vi "Polarity switch 2 channel.vi"() -> ()   [LabVIEW 2017]
uses:
  <vilib>/DAQmx/write.llb/DAQmx Write (Digital 1D Bool NChan 1Samp 1Line).vi
  <vilib>/DAQmx/read.llb/DAQmx Read (Analog DBL 1Chan 1Samp).vi
  <vilib>/DAQmx/miscellaneous.llb/DAQmx Fill In Error Info.vi
  <instrlib>/Keithley KE22xx Series/Keithley KE22xx Series.lvlib
  <instrlib>/Harvard Apparatus PHD Ultra Series/Harvard Apparatus PHD Ultra Series.lvlib
  <instrlib>/J-KEM Quad temperature control/J-KEM Quad temperature control.lvlib
panel:
  out "Channel 2 voltage (V)":dbl format="%0.3f"
  in  "Voltage control set 2 (V)":dbl=3.0 format="%.2f"
  in  "Channel 2 control":bool
  in  "Voltage control set 1 (V)":dbl=3.0 format="%.2f"
  in  "Channel 1 control":bool
  in  "Control voltage":bool
  out "Channel 1 voltage (V)":dbl format="%0.3f"
  in  "Voltage set 2 (V)":dbl=3.0 format="%.3f"
  in  "Enable Output 2":bool
  in  "DC channel 2":bool
  out "Current 2 (mA)":dbl
  out "Voltage 2 (V)":dbl
  in  "Read voltage 2":bool
  in  "DC channel 1":bool
  in  "Target wait time 2 (min)":dbl
  in  "Count down 2":bool
  in  "New sample 2":bool
  in  "base path 2":path
  in  "Sample name 2":string
  in  "Stop&Save 2":bool
  in  "Saving data 2":bool
  in  "Start switching 2":bool
  in  "Switching time 2 (s)":dbl
  out "Present 2 (s)":dbl caption="Present (s)"
  out "Current time 2":timestamp
  out "Sample waiting time 2 (min)":dbl
  out "Start time 2":timestamp
  in  "Timing 2":bool
  in  "Channel 2 SP (C)":dbl format="%#_13g"
  in  "Channel 1 SP (C)":dbl format="%#_13g"
  out "Temperature plot":T1(graph)
  in  "Channel 2":bool
  out "Channel 2 temperature (C)":dbl
  out "Channel 1 temperature (C)":dbl
  in  "Channel 1":bool
  in  "J-KEM COM":refnum<visa-resource-name>="COM15"
  in  "Pump COM 2":refnum<visa-resource-name>="COM12"
  in  "Flow Rate (ul/min) 2":dbl=5.0 format="%#.4f"
  in  "Set flow 2":bool
  out "Infusing  2":bool
  out "Withdrawing 2":bool
  out "Idle 2":bool
  in  "Status 2":bool
  in  "Start 2":bool
  in  "Stop 2":bool
  out "Volume 2":dbl
  out "Volume Units 2":u16(ring) items=["milliliters", "microliters", "nanoliters", "picoliters"]
  in  "Read volume&time 2":bool
  in  "Set pump 2":bool
  out "error out 2":errorcluster
  in  "Read volume&time 1":bool
  out "Volume Units 1":u16(ring) items=["milliliters", "microliters", "nanoliters", "picoliters"]
  out "Volume 1":dbl
  in  "Set pump 1":bool
  in  "Stop 1":bool
  in  "Start 1":bool
  in  "Status 1":bool
  out "Infusing 1":bool
  out "Withdrawing 1":bool
  out "Idle 1":bool
  in  "Set flow 1":bool
  in  "Flow Rate (ul/min)":dbl=5.0 format="%#.4f"
  in  "Pump COM 1":refnum<visa-resource-name>="COM4"
  in  "Target wait time 1 (min)":dbl
  in  "Count down 1":bool
  in  "New sample 1":bool
  in  "Sample name 1":string
  in  "base path 1":path
  in  "Stop&Save 1":bool
  in  "Saving data 1":bool
  out "Sample waiting time 1 (min)":dbl
  out "Current time 1":timestamp
  out "Start time 1":timestamp
  in  "Timing 1":bool
  in  "Read voltage 1":bool
  out "Electrolysis current Chart":cluster{dbl, dbl}(graph)
  out "Voltage 1 (V)":dbl
  out "Current 1 (mA)":dbl
  in  "Voltage set 1 (V)":dbl=3.0 min=0.0 format="%.3f"
  in  "Enable Output 1":bool
  in  "DC power supply":refnum<visa-resource-name>="USB0::0x05E6::0x2230::9101650::INSTR"
  out "Present 1 (s)":dbl caption="Present (s)"
  in  "stop":bool
  in  "Switching time 1 (s)":dbl
  in  "Start switching 1":bool
  # "Temperature control"
  # "General settings"
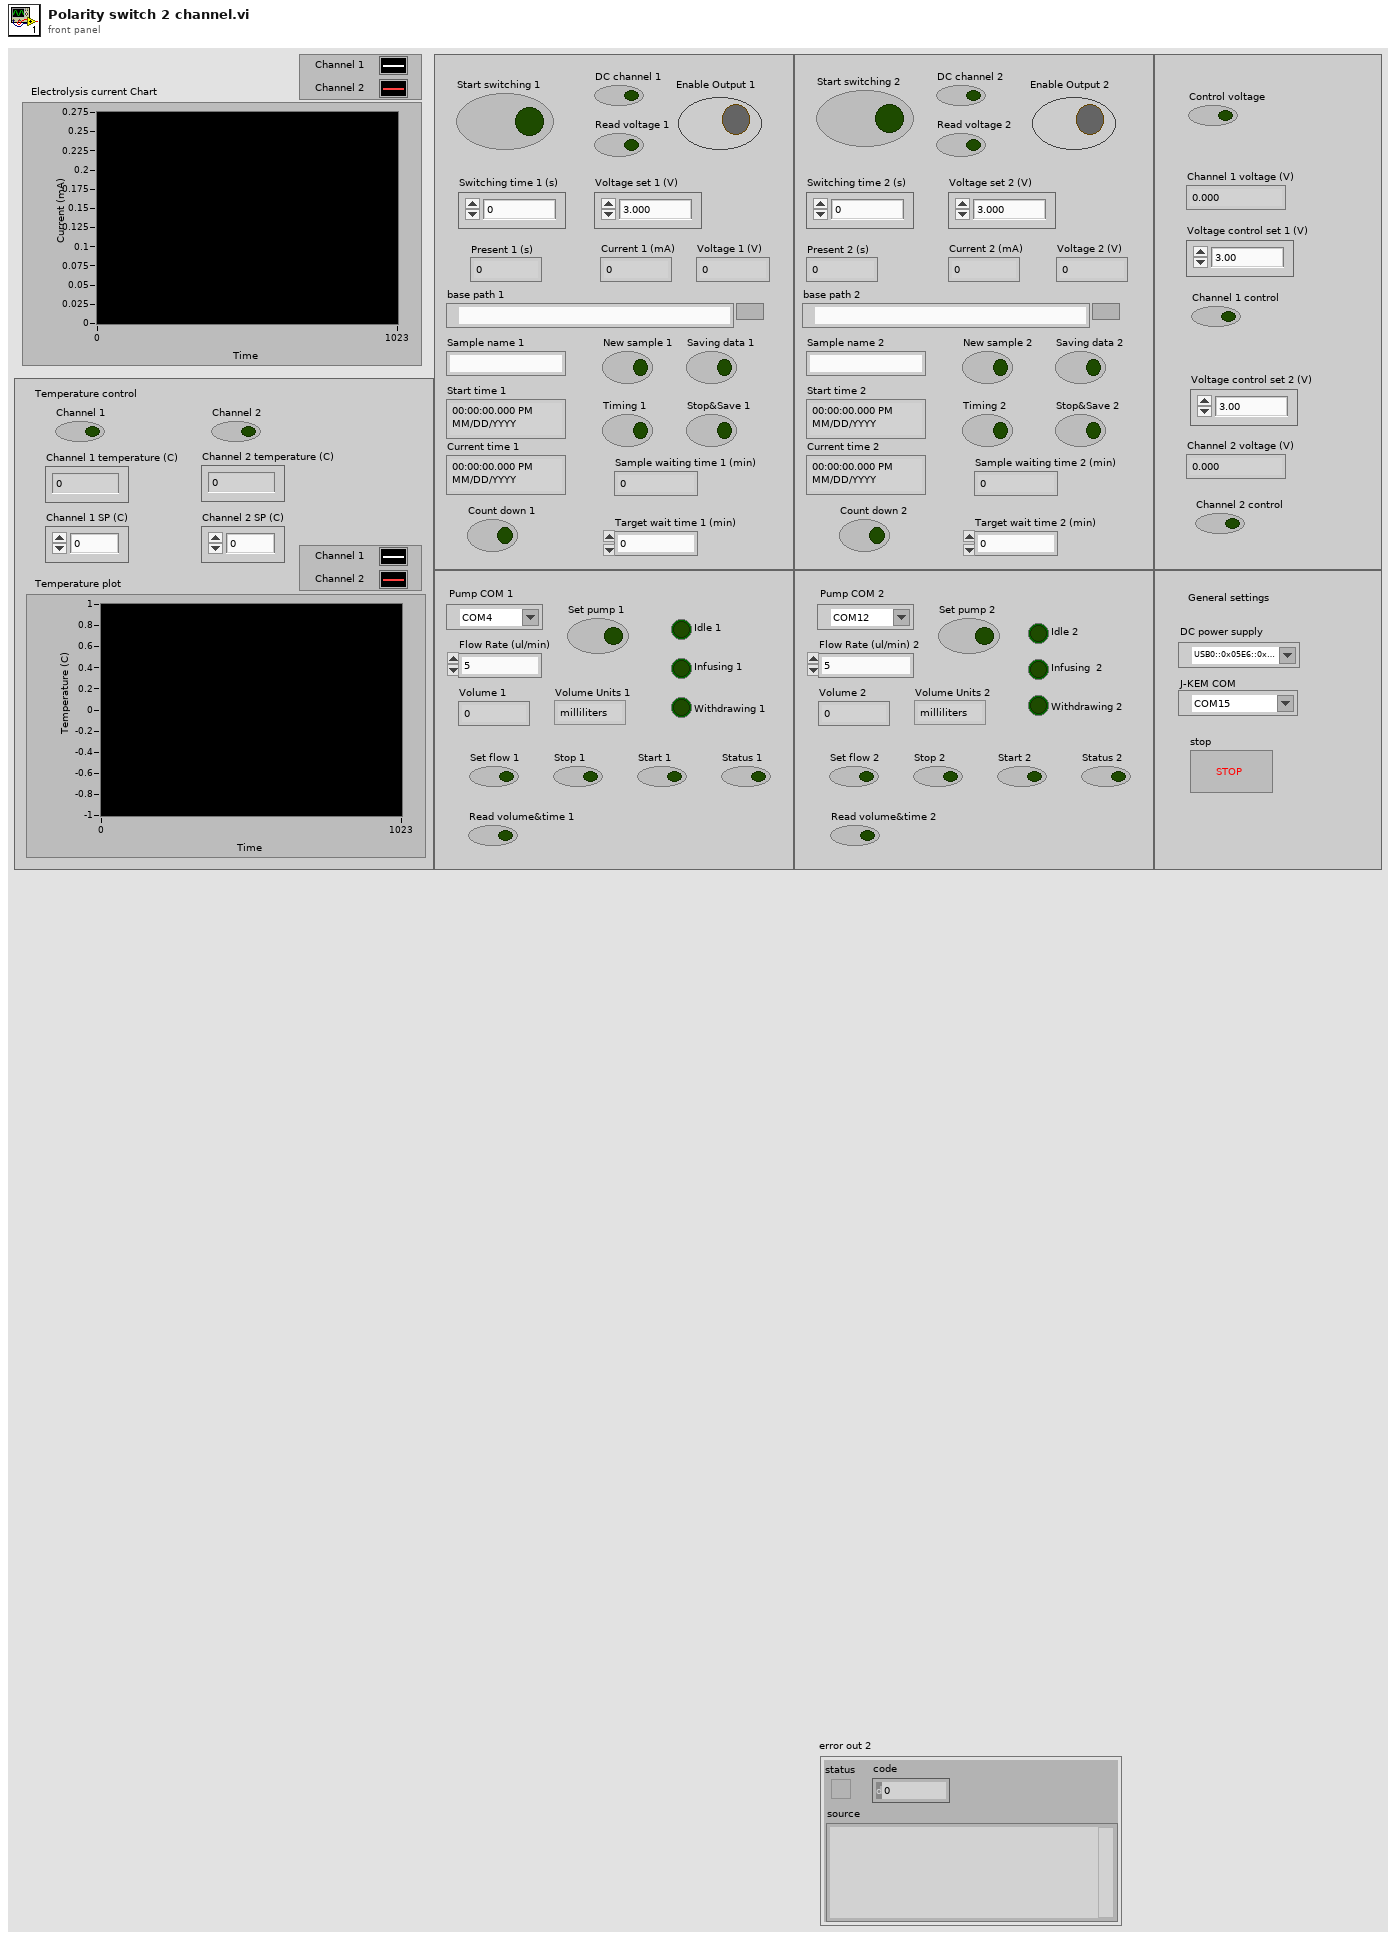
[diagram p1: front panel]
types:
  T1 = cluster{"Temperature (C)":dbl, "Temperature (C)":dbl}
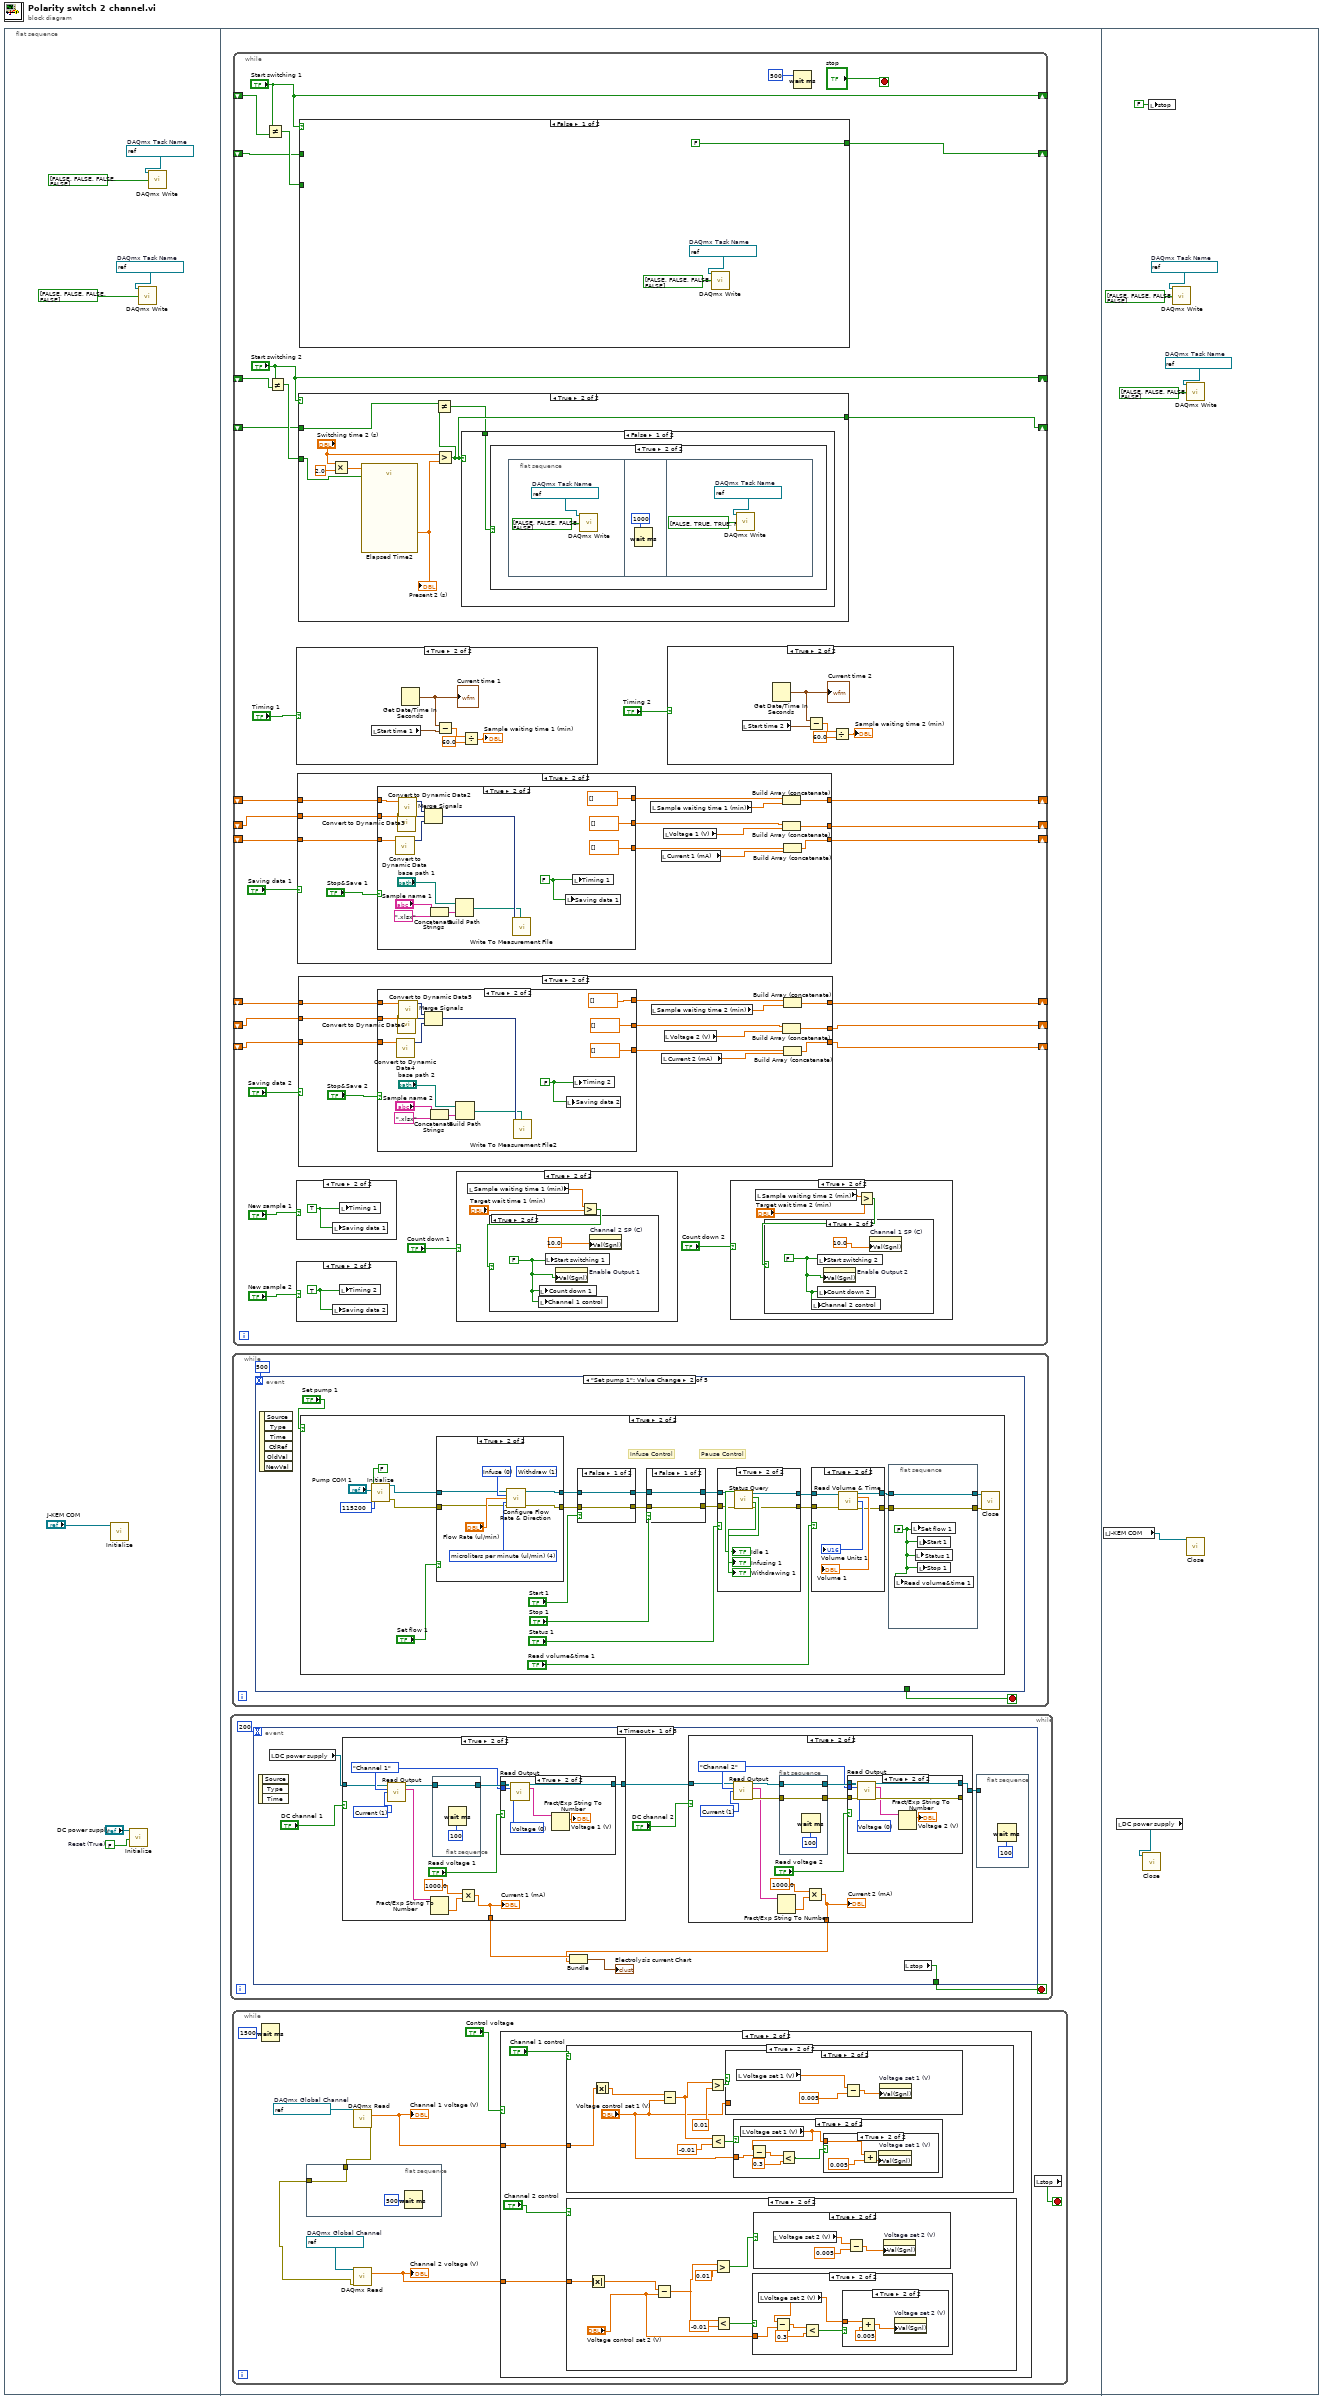
[diagram p0: block diagram]
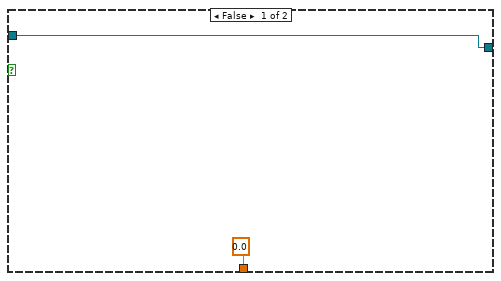
[diagram p11: hidden frame]
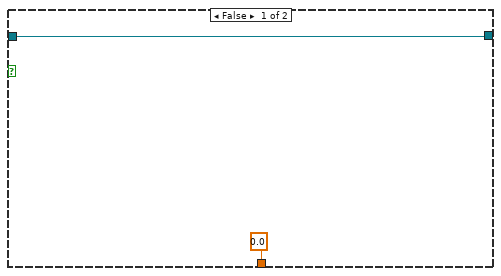
[diagram p13: hidden frame]
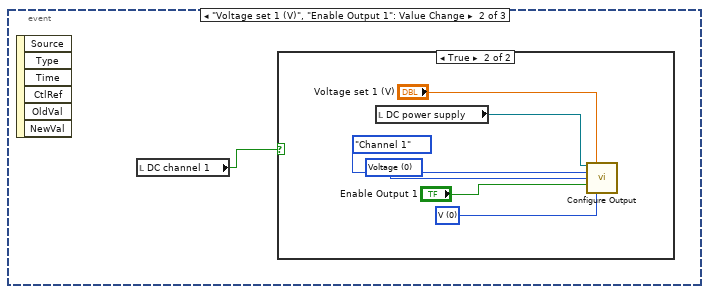
[diagram p15: hidden frame]
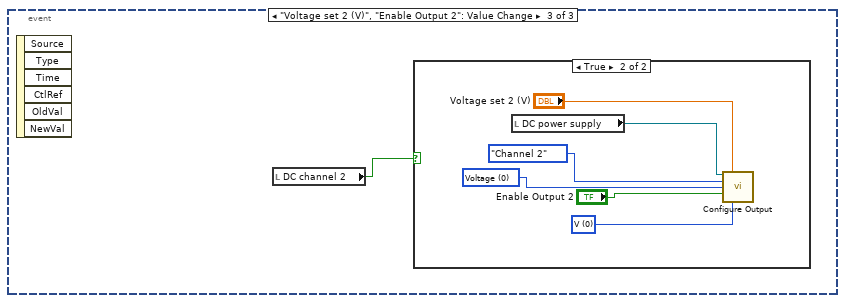
[diagram p17: hidden frame]
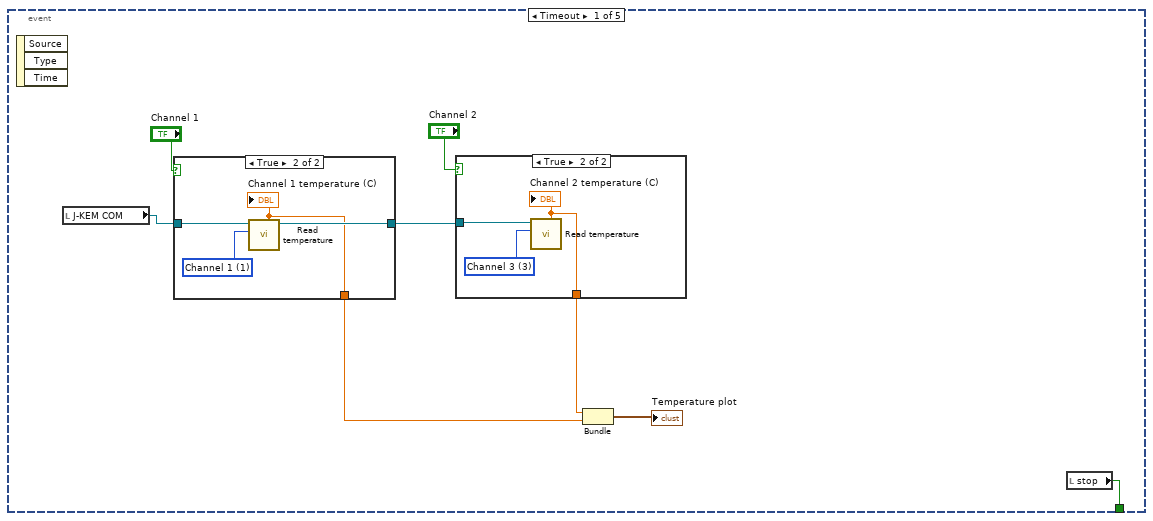
[diagram p19: hidden frame]
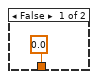
[diagram p20: hidden frame]
diagram:
  n1 = flat-sequence {
    frame #0 {
      w1 = refnum<k21> "Polarity swtich 2"  # DAQmx Task Name
      w5 = FALSE items=["OFF", "ON", "OFF", "ON"]  # Reset (True)
      w7 = refnum<k21> "Polarity switch 1"  # DAQmx Task Name
      n2 = call <instrlib>:"Initialize.vi"("VISA resource name"="J-KEM COM") -> ()  [unwired: 9 in, 2 out]
      n3 = call <instrlib>:"Initialize.vi"("Reset (True)"=w5, "VISA resource name"="DC power supply") -> ()  [unwired: 8 in, 2 out]
      n4 = call-poly <vilib>:"DAQmx Write.vi"("task/channels in"=w1, "data"=bool[] [FALSE, FALSE, FALSE, FALSE]) -> ()  [unwired: 11 in, 3 out]
      n5 = call-poly <vilib>:"DAQmx Write.vi"("task/channels in"=w7, "data"=bool[] [FALSE, FALSE, FALSE, FALSE]) -> ()  [unwired: 11 in, 3 out]
    }
    frame #1 {
      n6 = while {
        stop <- w62 stop-if-true
        n7 = event shown="[0] Timeout" {
          selector: _ -> [_ _ _]
          dyn-events: _ -> [_ _ _]
          timeout: 200 -> [_ _ _]
          tunnel: [w71 _ _] -> w62
          event Timeout {
            n8 = event-data() -> ()  [unwired: 1 in, 3 out]
            n9 = local read "DC power supply"() -> (w69:refnum<visa-resource-name>)
            n10 = case shown="True" "DC channel 1" {
              tunnel: w69 -> [w102 w105]
              tunnel: [w102 w104] -> w68
              tunnel: [0.0 w103] -> w66
              frame False {
              }
              frame True {
                w106 = u16 1 items=["Voltage", "Current", "Power"] ("Measurement Function (0:Voltage)")
                w108 = enum16{"Channel 1", "Channel 2", "Channel 3"}."Channel 1" ("Channel Select")
                n11 = call <instrlib>:"Read Output.vi"("VISA resource name"=w105, "Channel Select"=w108, "Measurement Function (0:Voltage)"=w106) -> ("VISA resource name out"=w112:refnum<visa-resource-name>, "Measurement"=w109:string)  [unwired: 10 in, 1 out]
                n12 = Fract/Exp String To Number(string=w109) -> (number=w110:dbl)  [unwired: 3 in, 1 out]
                n13 = flat-sequence {
                  tunnel: [w122] -> w111
                  tunnel: w112 -> [w122]
                  frame #0 {
                    n14 = Wait (ms)(milliseconds to wait=u32 100) -> ()  [unwired: 1 out]
                  }
                }
                n15 = Multiply(x=1000.0, y=w110) -> (x*y=w103:dbl)
                "Current 1 (mA)" <- w103
                n16 = case shown="True" "Read voltage 1" {
                  tunnel: [w114 w119] -> w104
                  tunnel: w111 -> [w114 w118]
                  tunnel: w108 -> [_ w117]
                  frame False {
                  }
                  frame True {
                    w120 = u16 0 items=["Voltage", "Current", "Power"] ("Measurement Function (0:Voltage)")
                    n17 = call <instrlib>:"Read Output.vi"("VISA resource name"=w118, "Channel Select"=w117, "Measurement Function (0:Voltage)"=w120) -> ("VISA resource name out"=w119:refnum<visa-resource-name>, "Measurement"=w115:string)  [unwired: 10 in, 1 out]
                    n18 = Fract/Exp String To Number(string=w115) -> (number=→"Voltage 1 (V)":dbl)  [unwired: 3 in, 1 out]
                  }
                }
              }
            }
            n19 = case shown="True" "DC channel 2" {
              tunnel: w68 -> [w73 w77]
              tunnel: [0.0 w76] -> w65
              tunnel: [w73 w75] -> w63
              frame False {
              }
              frame True {
                w78 = u16 1 items=["Voltage", "Current", "Power"] ("Measurement Function (0:Voltage)")
                w80 = enum16{"Channel 1", "Channel 2", "Channel 3"}."Channel 2" ("Channel Select")
                n20 = call <instrlib>:"Read Output.vi"("VISA resource name"=w77, "Channel Select"=w80, "Measurement Function (0:Voltage)"=w78) -> ("VISA resource name out"=w84:refnum<visa-resource-name>, "Measurement"=w81:string, "error out"=w86:errorcluster)  [unwired: 10 in]
                n21 = Fract/Exp String To Number(string=w81) -> (number=w82:dbl)  [unwired: 3 in, 1 out]
                n22 = flat-sequence {
                  tunnel: [w100] -> w83
                  tunnel: w84 -> [w100]
                  tunnel: [w99] -> w85
                  tunnel: w86 -> [w99]
                  frame #0 {
                    n23 = Wait (ms)(milliseconds to wait=u32 100) -> ()  [unwired: 1 out]
                  }
                }
                n24 = Multiply(x=1000.0, y=w82) -> (x*y=w76:dbl)
                "Current 2 (mA)" <- w76
                n25 = case shown="True" "Read voltage 2" {
                  tunnel: [w89 w96] -> w75
                  tunnel: [w88 w95] -> _
                  tunnel: w83 -> [w89 w94]
                  tunnel: w85 -> [w88 w93]
                  tunnel: w80 -> [_ w92]
                  frame False {
                  }
                  frame True {
                    w97 = u16 0 items=["Voltage", "Current", "Power"] ("Measurement Function (0:Voltage)")
                    n26 = call <instrlib>:"Read Output.vi"("VISA resource name"=w94, "Channel Select"=w92, "Measurement Function (0:Voltage)"=w97, "error in (no error)"=w93) -> ("VISA resource name out"=w96:refnum<visa-resource-name>, "Measurement"=w90:string, "error out"=w95:errorcluster)  [unwired: 9 in]
                    n27 = Fract/Exp String To Number(string=w90) -> (number=→"Voltage 2 (V)":dbl)  [unwired: 3 in, 1 out]
                  }
                }
              }
            }
            n28 = Bundle(w66, w65) -> (→"Electrolysis current Chart":cluster{dbl, dbl})  [unwired: 1 in]
            n29 = local read "stop"() -> (w71:bool)
            n30 = flat-sequence {
              tunnel: w63 -> [_]
              frame #0 {
                n31 = Wait (ms)(milliseconds to wait=u32 100) -> ()  [unwired: 1 out]
              }
            }
          }
          event "Voltage set 1 (V)", "Enable Output 1": Value Change {
            n32 = event-data() -> ()  [unwired: 1 in, 6 out]
            n33 = local read "DC channel 1"() -> (w123:bool)
            n34 = case shown="True" w123 {
              frame False {
              }
              frame True {
                w125 = u16 0 items=["Voltage", "Current"] ("Function(0:Voltage)")
                w124 = u16 0 items=["V", "mV", "kV", "A", "mA"] ("Unit(V)")
                n35 = local read "DC power supply"() -> (w127:refnum<visa-resource-name>)
                n36 = call <instrlib>:"Configure Output.vi"("VISA resource name"=w127, "Manual Range(0.00)"="Voltage set 1 (V)", "Channel Select"=enum16{"Channel 1", "Channel 2", "Channel 3"}."Channel 1", "Function(0:Voltage)"=w125, "Enable Output (T: Enable)"="Enable Output 1", "Unit(V)"=w124) -> ()  [unwired: 8 in, 2 out]
              }
            }
          }
          event "Voltage set 2 (V)", "Enable Output 2": Value Change {
            n37 = event-data() -> ()  [unwired: 1 in, 6 out]
            n38 = local read "DC channel 2"() -> (w130:bool)
            n39 = case shown="True" w130 {
              frame False {
              }
              frame True {
                w132 = u16 0 items=["Voltage", "Current"] ("Function(0:Voltage)")
                w131 = u16 0 items=["V", "mV", "kV", "A", "mA"] ("Unit(V)")
                n40 = local read "DC power supply"() -> (w134:refnum<visa-resource-name>)
                n41 = call <instrlib>:"Configure Output.vi"("VISA resource name"=w134, "Manual Range(0.00)"="Voltage set 2 (V)", "Channel Select"=enum16{"Channel 1", "Channel 2", "Channel 3"}."Channel 2", "Function(0:Voltage)"=w132, "Enable Output (T: Enable)"="Enable Output 2", "Unit(V)"=w131) -> ()  [unwired: 8 in, 2 out]
              }
            }
          }
        }
      }
      n42 = while {
        stop <- w137 stop-if-true
        n43 = event shown="[1] \"Set pump 1\": Value Change" {
          selector: _ -> [_ _ _ _ _]
          dyn-events: _ -> [_ _ _ _ _]
          timeout: 500 -> [_ _ _ _ _]
          tunnel: [w139 _ _ _ _] -> w137
          event Timeout {
            n44 = event-data() -> ()  [unwired: 1 in, 3 out]
            n45 = local read "J-KEM COM"() -> (w145:refnum<visa-resource-name>)
            n46 = case shown="True" "Channel 1" {
              tunnel: w145 -> [w152 w156]
              tunnel: [w152 w154] -> w144
              tunnel: [0.0 ("Temperature (C)") w153] -> w142
              frame False {
              }
              frame True {
                w155 = u16 1 items=["Channel 1"=1, "Channel 2"=2, "Channel 3"=3, "Channel 4"=4] ("Channel")
                n47 = call <instrlib>:"Read temperature.vi"("Channel"=w155, "VISA resource"=w156) -> ("Temperature (C)"=w153:dbl, "VISA resource"=w154:refnum<visa-resource-name>)  [unwired: 7 in, 1 out]
                "Channel 1 temperature (C)" <- w153
              }
            }
            n48 = case shown="True" "Channel 2" {
              tunnel: w144 -> [_ w150]
              tunnel: [0.0 ("Temperature (C)") w148] -> w141
              frame False {
              }
              frame True {
                w149 = u16 3 items=["Channel 1"=1, "Channel 2"=2, "Channel 3"=3, "Channel 4"=4] ("Channel")
                n49 = call <instrlib>:"Read temperature.vi"("Channel"=w149, "VISA resource"=w150) -> ("Temperature (C)"=w148:dbl)  [unwired: 7 in, 2 out]
                "Channel 2 temperature (C)" <- w148
              }
            }
            n50 = Bundle("Temperature (C)"=w141, "Temperature (C)"=w142) -> (→"Temperature plot":T1)  [unwired: 1 in]
            n51 = local read "stop"() -> (w139:bool)
          }
          event "Set pump 1": Value Change {
            n52 = event-data() -> ()  [unwired: 1 in, 6 out]
            n53 = case shown="True" "Set pump 1" {
              frame False {
              }
              frame True {
                w178 = u32 115200 items=["9600"=9600, "19200"=19200, "38400"=38400, "57600"=57600, "115200"=115200] ("Baud Rate (115200)")
                # "Pause Control"
                # "Infuse Control"
                n54 = call <instrlib>:"Initialize.vi"("ID Query (True)"=FALSE, "Baud Rate (115200)"=w178, "VISA resource name"="Pump COM 1") -> ("error out"=w173:errorcluster, "VISA resource name out"=w174:refnum<visa-resource-name>)  [unwired: 7 in]
                n55 = case shown="True" "Set flow 1" {
                  tunnel: w174 -> [w201 w205]
                  tunnel: w173 -> [w200 w204]
                  tunnel: [w201 w203] -> w172
                  tunnel: [w200 w202] -> w171
                  frame False {
                  }
                  frame True {
                    w206 = u32 4 items=["milliliters per hour (ml/hr)", "milliliters per minute (ml/min)", "milliliters per second (ml/sec)", "microliters per hour (ul/hr)", "microliters per minute (ul/min)", "microliters per second (ul/sec)", "nanoliters per hour (nl/hr)", "nanoliters per minute (nl/min)", "nanoliters per second (nl/sec)", "picoliters per hour (pl/hr)", "picoliters per minute (pl/min)", "picoliters per second (pl/sec)"] ("Flow Rate Units")
                    w208 = u16 0 items=["Infuse", "Withdraw"] ("Pump Method (0:Infuse)")
                    (unwired) u16 1 items=["Infuse", "Withdraw"] ("Pump Method (0:Infuse)")
                    n56 = call <instrlib>:"Configure Flow Rate & Direction.vi"("VISA resource name"=w205, "Pump Direction (0:Infuse)"=w208, "Flow Rate (5.00)"="Flow Rate (ul/min)", "Flow Rate Units (1:ml/min)"=w206, "error in (no error)"=w204) -> ("VISA resource name out"=w203:refnum<visa-resource-name>, "error out"=w202:errorcluster)  [unwired: 9 in]
                  }
                }
                n57 = case shown="False" "Start 1" {
                  tunnel: [w216 w221] -> w177
                  tunnel: [w215 w220] -> w176
                  tunnel: w172 -> [w216 w218]
                  tunnel: w171 -> [w215 w217]
                  frame False {
                  }
                  frame True {
                    w219 = u16 0 items=["Infuse", "Withdraw"] ("Run Method (0:Infuse)")
                    n58 = call <instrlib>:"Start Pump.vi"("error in (no error)"=w217, "Run Direction (0:Infuse)"=w219, "VISA resource name"=w218) -> ("error out"=w220:errorcluster, "VISA resource name out"=w221:refnum<visa-resource-name>)  [unwired: 7 in]
                  }
                }
                n59 = case shown="False" "Stop 1" {
                  tunnel: w177 -> [w210 w214]
                  tunnel: w176 -> [w209 w213]
                  tunnel: [w210 w212] -> w170
                  tunnel: [w209 w211] -> w169
                  frame False {
                  }
                  frame True {
                    n60 = call <instrlib>:"Stop Pump.vi"("error in (no error)"=w213, "VISA resource name"=w214) -> ("error out"=w211:errorcluster, "VISA resource name out"=w212:refnum<visa-resource-name>)  [unwired: 8 in]
                  }
                }
                n61 = case shown="True" "Status 1" {
                  tunnel: w170 -> [w192 w196]
                  tunnel: w169 -> [w191 w195]
                  tunnel: [w192 w194] -> w162
                  tunnel: [w191 w193] -> w161
                  frame False {
                  }
                  frame True {
                    n62 = call <instrlib>:"Status Query.vi"("error in (no error)"=w195, "VISA resource name"=w196) -> ("error out"=w193:errorcluster, "Withdrawing"=→"Withdrawing 1":bool, "Infusing"=→"Infusing 1":bool, "VISA resource name out"=w194:refnum<visa-resource-name>, "Idle"=→"Idle 1":bool)  [unwired: 4 in, 1 out]
                  }
                }
                n63 = case shown="True" "Read volume&time 1" {
                  tunnel: w162 -> [w181 w187]
                  tunnel: w161 -> [w180 w186]
                  tunnel: [w181 w183] -> w160
                  tunnel: [w180 w182] -> w159
                  frame False {
                  }
                  frame True {
                    n64 = call <instrlib>:"Read Volume & Time .vi"("VISA resource name"=w187, "error in (no error)"=w186) -> ("VISA resource name out"=w183:refnum<visa-resource-name>, "Volume"=→"Volume 1":dbl, "Volume Units"=→"Volume Units 1":u16, "error out"=w182:errorcluster)  [unwired: 8 in, 2 out]
                  }
                }
                n65 = flat-sequence {
                  tunnel: w160 -> [w189]
                  tunnel: [w190] -> w165
                  tunnel: w159 -> [w190]
                  tunnel: [w189] -> w164
                  frame #0 {
                    w188 = FALSE
                    n66 = local write "Read volume&time 1"(w188) -> ()
                    n67 = local write "Set flow 1"(w188) -> ()
                    n68 = local write "Status 1"(w188) -> ()
                    n69 = local write "Start 1"(w188) -> ()
                    n70 = local write "Stop 1"(w188) -> ()
                  }
                }
                n71 = call <instrlib>:"Close.vi"("error in (no error)"=w165, "VISA resource name"=w164) -> ()  [unwired: 9 in, 1 out]
              }
            }
          }
          event "Set pump 2": Value Change {
            n72 = event-data() -> ()  [unwired: 1 in, 6 out]
            n73 = case shown="True" "Set pump 2" {
              frame False {
              }
              frame True {
                w243 = u32 115200 items=["9600"=9600, "19200"=19200, "38400"=38400, "57600"=57600, "115200"=115200] ("Baud Rate (115200)")
                # "Pause Control"
                # "Infuse Control"
                n74 = call <instrlib>:"Initialize.vi"("ID Query (True)"=FALSE, "Baud Rate (115200)"=w243, "VISA resource name"="Pump COM 2") -> ("error out"=w238:errorcluster, "VISA resource name out"=w239:refnum<visa-resource-name>)  [unwired: 7 in]
                "error out 2" <- w238
                n75 = case shown="True" "Set flow 2" {
                  tunnel: w239 -> [w266 w270]
                  tunnel: w238 -> [w265 w269]
                  tunnel: [w266 w268] -> w237
                  tunnel: [w265 w267] -> w236
                  frame False {
                  }
                  frame True {
                    w271 = u32 4 items=["milliliters per hour (ml/hr)", "milliliters per minute (ml/min)", "milliliters per second (ml/sec)", "microliters per hour (ul/hr)", "microliters per minute (ul/min)", "microliters per second (ul/sec)", "nanoliters per hour (nl/hr)", "nanoliters per minute (nl/min)", "nanoliters per second (nl/sec)", "picoliters per hour (pl/hr)", "picoliters per minute (pl/min)", "picoliters per second (pl/sec)"] ("Flow Rate Units")
                    w273 = u16 0 items=["Infuse", "Withdraw"] ("Pump Method (0:Infuse)")
                    (unwired) u16 1 items=["Infuse", "Withdraw"] ("Pump Method (0:Infuse)")
                    n76 = call <instrlib>:"Configure Flow Rate & Direction.vi"("VISA resource name"=w270, "Pump Direction (0:Infuse)"=w273, "Flow Rate (5.00)"="Flow Rate (ul/min) 2", "Flow Rate Units (1:ml/min)"=w271, "error in (no error)"=w269) -> ("VISA resource name out"=w268:refnum<visa-resource-name>, "error out"=w267:errorcluster)  [unwired: 9 in]
                  }
                }
                n77 = case shown="False" "Start 2" {
                  tunnel: [w281 w286] -> w242
                  tunnel: [w280 w285] -> w241
                  tunnel: w237 -> [w281 w283]
                  tunnel: w236 -> [w280 w282]
                  frame False {
                  }
                  frame True {
                    w284 = u16 0 items=["Infuse", "Withdraw"] ("Run Method (0:Infuse)")
                    n78 = call <instrlib>:"Start Pump.vi"("error in (no error)"=w282, "Run Direction (0:Infuse)"=w284, "VISA resource name"=w283) -> ("error out"=w285:errorcluster, "VISA resource name out"=w286:refnum<visa-resource-name>)  [unwired: 7 in]
                  }
                }
                n79 = case shown="False" "Stop 2" {
                  tunnel: w242 -> [w275 w279]
                  tunnel: w241 -> [w274 w278]
                  tunnel: [w275 w277] -> w235
                  tunnel: [w274 w276] -> w234
                  frame False {
                  }
                  frame True {
                    n80 = call <instrlib>:"Stop Pump.vi"("error in (no error)"=w278, "VISA resource name"=w279) -> ("error out"=w276:errorcluster, "VISA resource name out"=w277:refnum<visa-resource-name>)  [unwired: 8 in]
                  }
                }
                n81 = case shown="True" "Status 2" {
                  tunnel: w235 -> [w257 w261]
                  tunnel: w234 -> [w256 w260]
                  tunnel: [w257 w259] -> w227
                  tunnel: [w256 w258] -> w226
                  frame False {
                  }
                  frame True {
                    n82 = call <instrlib>:"Status Query.vi"("error in (no error)"=w260, "VISA resource name"=w261) -> ("error out"=w258:errorcluster, "Withdrawing"=→"Withdrawing 2":bool, "Infusing"=→"Infusing  2":bool, "VISA resource name out"=w259:refnum<visa-resource-name>, "Idle"=→"Idle 2":bool)  [unwired: 4 in, 1 out]
                  }
                }
                n83 = case shown="True" "Read volume&time 2" {
                  tunnel: w227 -> [w246 w252]
                  tunnel: w226 -> [w245 w251]
                  tunnel: [w246 w248] -> w225
                  tunnel: [w245 w247] -> w224
                  frame False {
                  }
                  frame True {
                    n84 = call <instrlib>:"Read Volume & Time .vi"("VISA resource name"=w252, "error in (no error)"=w251) -> ("VISA resource name out"=w248:refnum<visa-resource-name>, "Volume"=→"Volume 2":dbl, "Volume Units"=→"Volume Units 2":u16, "error out"=w247:errorcluster)  [unwired: 8 in, 2 out]
                  }
                }
                n85 = flat-sequence {
                  tunnel: w225 -> [w254]
                  tunnel: [w255] -> w230
                  tunnel: w224 -> [w255]
                  tunnel: [w254] -> w229
                  frame #0 {
                    w253 = FALSE
                    n86 = local write "Read volume&time 2"(w253) -> ()
                    n87 = local write "Set flow 2"(w253) -> ()
                    n88 = local write "Status 2"(w253) -> ()
                    n89 = local write "Start 2"(w253) -> ()
                    n90 = local write "Stop 2"(w253) -> ()
                  }
                }
                n91 = call <instrlib>:"Close.vi"("error in (no error)"=w230, "VISA resource name"=w229) -> ()  [unwired: 9 in, 1 out]
              }
            }
          }
          event "Channel 1 SP (C)": Value Change {
            n92 = event-data() -> ()  [unwired: 1 in, 6 out]
            n93 = local read "Channel 1"() -> (w287:bool)
            n94 = case shown="True" w287 {
              frame False {
              }
              frame True {
                w289 = u16 1 items=["Channel 1"=1, "Channel 2"=2, "Channel 3"=3, "Channel 4"=4] ("Channel")
                n95 = local read "J-KEM COM"() -> (w290:refnum<visa-resource-name>)
                n96 = call <instrlib>:"Set SP.vi"("Set point (C)"="Channel 1 SP (C)", "Channel"=w289, "VISA resource name"=w290) -> ()  [unwired: 6 in, 3 out]
                n97 = Wait (ms)(milliseconds to wait=u32 1000) -> ()  [unwired: 1 out]
              }
            }
          }
          event "Channel 2 SP (C)": Value Change {
            n98 = event-data() -> ()  [unwired: 1 in, 6 out]
            n99 = local read "Channel 2"() -> (w292:bool)
            n100 = case shown="True" w292 {
              frame False {
              }
              frame True {
                w294 = u16 3 items=["Channel 1"=1, "Channel 2"=2, "Channel 3"=3, "Channel 4"=4] ("Channel")
                n101 = local read "J-KEM COM"() -> (w296:refnum<visa-resource-name>)
                n102 = call <instrlib>:"Set SP.vi"("Set point (C)"="Channel 2 SP (C)", "Channel"=w294, "VISA resource name"=w296) -> ()  [unwired: 6 in, 3 out]
                n103 = Wait (ms)(milliseconds to wait=u32 1000) -> ()  [unwired: 1 out]
              }
            }
          }
        }
      }
      n104 = while {
        stop <- w16 stop-if-true
        w11 = refnum<k21> "USB-6221 ai1"  # DAQmx Global Channel
        w13 = refnum<k21> "USB-6221 ai0"  # DAQmx Global Channel
        n105 = Wait (ms)(milliseconds to wait=u32 1500) -> ()  [unwired: 1 out]
        n106 = flat-sequence {
          tunnel: w10 -> [w18]
          tunnel: [w18] -> w9
          frame #0 {
            n107 = Wait (ms)(milliseconds to wait=u32 500) -> ()  [unwired: 1 out]
          }
        }
        n108 = call-poly <vilib>:"DAQmx Read.vi"("task/channels in"=w13) -> ("data"=w12:dbl, "error out"=w10:errorcluster)  [unwired: 12 in, 1 out]
        "Channel 1 voltage (V)" <- w12
        n109 = call-poly <vilib>:"DAQmx Read.vi"("task/channels in"=w11, "error in"=w9) -> ("data"=w8:dbl)  [unwired: 11 in, 2 out]
        "Channel 2 voltage (V)" <- w8
        n110 = case shown="True" "Control voltage" {
          tunnel: w12 -> [_ w21]
          tunnel: w8 -> [_ w19]
          frame False {
          }
          frame True {
            n111 = case shown="True" "Channel 1 control" {
              tunnel: w21 -> [_ w43]
              frame False {
              }
              frame True {
                n112 = Absolute Value(x=w43) -> (abs(x)=w49:dbl)
                n113 = Subtract(x=w49, y="Voltage control set 1 (V)") -> (x-y=w46:dbl)
                n114 = Greater?(x=w46, y=0.01) -> (0:w47:bool)
                n115 = Less?(x=w46, y=-0.01) -> (x < y?=w44:bool)
                n116 = case shown="True" w47 {
                  tunnel: "Voltage control set 1 (V)" -> [_ _]
                  frame False {
                  }
                  frame True {
                    n117 = local read "Voltage set 1 (V)"() -> (w60:dbl)
                    n118 = Subtract(x=w60, y=0.005) -> (x-y=w58:dbl)
                    n119 = property on="Voltage set 1 (V)" class="DigNum (strict)"("Val(Sgnl)"=w58) -> ()  [unwired: 2 in, 2 out]
                  }
                }
                n120 = case shown="True" w44 {
                  tunnel: "Voltage control set 1 (V)" -> [_ w54]
                  frame False {
                  }
                  frame True {
                    n121 = local read "Voltage set 1 (V)"() -> (w53:dbl)
                    n122 = Subtract(x=w53, y=w54) -> (x-y=w50:dbl)
                    n123 = Less?(x=w50, y=0.3) -> (x < y?=w51:bool)
                    n124 = case shown="True" w51 {
                      tunnel: w53 -> [_ w55]
                      frame False {
                      }
                      frame True {
                        n125 = Add(x=w55, y=0.005) -> (x+y=w56:dbl)
                        n126 = property on="Voltage set 1 (V)" class="DigNum (strict)"("Val(Sgnl)"=w56) -> ()  [unwired: 2 in, 2 out]
                      }
                    }
                  }
                }
              }
            }
            n127 = case shown="True" "Channel 2 control" {
              tunnel: w19 -> [_ w30]
              frame False {
              }
              frame True {
                n128 = Absolute Value(x=w30) -> (abs(x)=w29:dbl)
                n129 = Subtract(x=w29, y="Voltage control set 2 (V)") -> (x-y=w26:dbl)
                n130 = Greater?(x=w26, y=0.01) -> (0:w25:bool)
                n131 = Less?(x=w26, y=-0.01) -> (x < y?=w24:bool)
                n132 = case shown="True" w24 {
                  tunnel: "Voltage control set 2 (V)" -> [_ w33]
                  frame False {
                  }
                  frame True {
                    n133 = local read "Voltage set 2 (V)"() -> (w32:dbl)
                    n134 = Subtract(x=w32, y=w33) -> (x-y=w35:dbl)
                    n135 = Less?(x=w35, y=0.3) -> (x < y?=w31:bool)
                    n136 = case shown="True" w31 {
                      tunnel: w32 -> [_ w36]
                      frame False {
                      }
                      frame True {
                        n137 = Add(x=w36, y=0.005) -> (x+y=w37:dbl)
                        n138 = property on="Voltage set 2 (V)" class="DigNum (strict)"("Val(Sgnl)"=w37) -> ()  [unwired: 2 in, 2 out]
                      }
                    }
                  }
                }
                n139 = case shown="True" w25 {
                  frame False {
                  }
                  frame True {
                    n140 = local read "Voltage set 2 (V)"() -> (w40:dbl)
                    n141 = Subtract(x=w40, y=0.005) -> (x-y=w39:dbl)
                    n142 = property on="Voltage set 2 (V)" class="DigNum (strict)"("Val(Sgnl)"=w39) -> ()  [unwired: 2 in, 2 out]
                  }
                }
              }
            }
          }
        }
        n143 = local read "stop"() -> (w16:bool)
      }
      n144 = while {
        shift-right: ["Start switching 1"] -> _
        shift-left: _ -> [w327]
        shift-right: [w325] -> _
        shift-left: _ -> [w324]
        shift-right: [w319] -> _
        shift-left: _ -> [w317]
        shift-right: [w318] -> _
        shift-left: _ -> [w316]
        shift-right: ["Start switching 2"] -> _
        shift-left: _ -> [w311]
        shift-right: [w309] -> _
        shift-left: _ -> [w308]
        shift-right: [w307] -> _
        shift-left: _ -> [w306]
        shift-right: [w304] -> _
        shift-left: _ -> [w301]
        shift-right: [w303] -> _
        shift-left: _ -> [w300]
        shift-right: [w302] -> _
        shift-left: _ -> [w299]
        stop <- "stop" stop-if-true
        n145 = Not Equal?(x="Start switching 1", y=w327) -> (x != y?=w326:bool)
        n146 = Not Equal?(x="Start switching 2", y=w311) -> (x != y?=w310:bool)
        n147 = case shown="True" "Timing 1" {
          frame False {
            n148 = Get Date/Time In Seconds() -> (seconds since 1Jan1904=→"Start time 1":timestamp)
          }
          frame True {
            n149 = local read "Start time 1"() -> (w444:timestamp)
            n150 = Get Date/Time In Seconds() -> (seconds since 1Jan1904=w445:timestamp)
            "Current time 1" <- w445
            n151 = Subtract(x=w445, y=w444) -> (x-y=w442:dbl)
            n152 = Divide(x=w442, y=60.0) -> (x/y=→"Sample waiting time 1 (min)":dbl)
          }
        }
        n153 = case shown="True" "New sample 1" {
          frame False {
          }
          frame True {
            w404 = TRUE ("Timing")
            n154 = local write "Saving data 1"(w404) -> ()
            n155 = local write "Timing 1"(w404) -> ()
          }
        }
        n156 = case shown="True" "New sample 2" {
          frame False {
          }
          frame True {
            w334 = TRUE ("Timing")
            n157 = local write "Saving data 2"(w334) -> ()
            n158 = local write "Timing 2"(w334) -> ()
          }
        }
        n159 = case shown="True" "Saving data 1" {
          tunnel: [dbl[] [] w420] -> w319
          tunnel: [dbl[] [] w412] -> w318
          tunnel: w317 -> [_ w415]
          tunnel: w316 -> [_ w414]
          tunnel: [dbl[] [] w409] -> w307
          tunnel: w306 -> [_ w408]
          frame False {
          }
          frame True {
            n160 = case shown="True" "Stop&Save 1" {
              tunnel: [w423 dbl[] []] -> w416
              tunnel: w415 -> [w423 w438]
              tunnel: [w421 dbl[] []] -> w410
              tunnel: w414 -> [w422 w439]
              tunnel: [w422 dbl[] []] -> w411
              tunnel: w408 -> [w421 w426]
              frame False {
              }
              frame True {
                w428 = FALSE ("Timing")
                n161 = call "Convert to Dynamic Data"("Array"=w439) -> ("Dynamic Data Type"=w424:dynamicdata)  [unwired: 3 in]
                n162 = call "Convert to Dynamic Data3"("Array"=w426) -> ("Dynamic Data Type"=w425:dynamicdata)  [unwired: 3 in]
                n163 = call "Convert to Dynamic Data2"("Array"=w438) -> ("Dynamic Data Type"=w437:dynamicdata)  [unwired: 3 in]
                n164 = Merge Signals(w437, w425, w424) -> (w436:dynamicdata)
                n165 = Concatenate Strings("Sample name 1", ".xlsx" ("string")) -> (w430:string)
                n166 = Build Path(base path="base path 1", name or relative path=w430) -> (appended path=w434:path)
                n167 = call "Write To Measurement File"("Signals"=w436, "Filename"=w434) -> ()  [unwired: 15 in, 3 out]
                n168 = local write "Saving data 1"(w428) -> ()
                n169 = local write "Timing 1"(w428) -> ()
              }
            }
            n170 = local read "Sample waiting time 1 (min)"() -> (w419:dbl)
            n171 = local read "Current 1 (mA)"() -> (w418:dbl)
            n172 = local read "Voltage 1 (V)"() -> (w413:dbl)
            n173 = Build Array (concatenate)(w410, w413) -> (w409:dbl[])
            n174 = Build Array (concatenate)(w416, w419) -> (w420:dbl[])
            n175 = Build Array (concatenate)(w411, w418) -> (w412:dbl[])
          }
        }
        n176 = case shown="True" "Saving data 2" {
          tunnel: [dbl[] [] w350] -> w304
          tunnel: [dbl[] [] w342] -> w302
          tunnel: w301 -> [_ w345]
          tunnel: w299 -> [_ w344]
          tunnel: [dbl[] [] w339] -> w303
          tunnel: w300 -> [_ w338]
          frame False {
          }
          frame True {
            n177 = case shown="True" "Stop&Save 2" {
              tunnel: [w353 dbl[] []] -> w346
              tunnel: w345 -> [w353 w368]
              tunnel: [w351 dbl[] []] -> w340
              tunnel: w344 -> [w352 w369]
              tunnel: [w352 dbl[] []] -> w341
              tunnel: w338 -> [w351 w356]
              frame False {
              }
              frame True {
                w358 = FALSE ("Timing")
                n178 = call "Convert to Dynamic Data4"("Array"=w369) -> ("Dynamic Data Type"=w354:dynamicdata)  [unwired: 3 in]
                n179 = call "Convert to Dynamic Data6"("Array"=w356) -> ("Dynamic Data Type"=w355:dynamicdata)  [unwired: 3 in]
                n180 = call "Convert to Dynamic Data5"("Array"=w368) -> ("Dynamic Data Type"=w367:dynamicdata)  [unwired: 3 in]
                n181 = Merge Signals(w367, w355, w354) -> (w366:dynamicdata)
                n182 = Concatenate Strings("Sample name 2", ".xlsx" ("string")) -> (w360:string)
                n183 = Build Path(base path="base path 2", name or relative path=w360) -> (appended path=w364:path)
                n184 = call "Write To Measurement File2"("Signals"=w366, "Filename"=w364) -> ()  [unwired: 15 in, 3 out]
                n185 = local write "Saving data 2"(w358) -> ()
                n186 = local write "Timing 2"(w358) -> ()
              }
            }
            n187 = local read "Sample waiting time 2 (min)"() -> (w349:dbl)
            n188 = local read "Current 2 (mA)"() -> (w348:dbl)
            n189 = local read "Voltage 2 (V)"() -> (w343:dbl)
            n190 = Build Array (concatenate)(w340, w343) -> (w339:dbl[])
            n191 = Build Array (concatenate)(w346, w349) -> (w350:dbl[])
            n192 = Build Array (concatenate)(w341, w348) -> (w342:dbl[])
          }
        }
        n193 = case shown="True" "Start switching 2" {
          tunnel: w310 -> [_ w373]
          tunnel: [FALSE w377] -> w309
          tunnel: w308 -> [_ w376]
          frame False {
            w370 = refnum<k21> "Polarity swtich 2"  # DAQmx Task Name
            n194 = call-poly <vilib>:"DAQmx Write.vi"("task/channels in"=w370, "data"=bool[] [FALSE, FALSE, FALSE, FALSE]) -> ()  [unwired: 11 in, 3 out]
          }
          frame True {
            n195 = Multiply(x="Switching time 2 (s)", y=2.0) -> (x*y=w379:dbl)
            n196 = call "Elapsed Time2"("Time Target (s)"=w379, "Reset"=w373) -> ("Elapsed Time (s)"=w374:dbl)  [unwired: 10 in, 7 out]
            "Present 2 (s)" <- w374
            n197 = Greater?(x="Switching time 2 (s)", y=w374) -> (0:w377:bool)
            n198 = Not Equal?(x=w376, y=w377) -> (x != y?=w375:bool)
            n199 = case shown="False" w377 {
              tunnel: w375 -> [w381 w387]
              frame False {
                n200 = case shown="True" w381 {
                  frame False {
                  }
                  frame True {
                    n201 = flat-sequence {
                      frame #0 {
                        w383 = refnum<k21> "Polarity swtich 2"  # DAQmx Task Name
                        n202 = call-poly <vilib>:"DAQmx Write.vi"("task/channels in"=w383, "data"=bool[] [FALSE, FALSE, FALSE, FALSE]) -> ()  [unwired: 11 in, 3 out]
                      }
                      frame #1 {
                        n203 = Wait (ms)(milliseconds to wait=u32 1000) -> ()  [unwired: 1 out]
                      }
                      frame #2 {
                        w385 = refnum<k21> "Polarity swtich 2"  # DAQmx Task Name
                        n204 = call-poly <vilib>:"DAQmx Write.vi"("task/channels in"=w385, "data"=bool[] [FALSE, TRUE, TRUE, FALSE]) -> ()  [unwired: 11 in, 3 out]
                      }
                    }
                  }
                }
              }
              frame True {
                n205 = case shown="True" w387 {
                  frame False {
                  }
                  frame True {
                    n206 = flat-sequence {
                      frame #0 {
                        w389 = refnum<k21> "Polarity swtich 2"  # DAQmx Task Name
                        n207 = call-poly <vilib>:"DAQmx Write.vi"("task/channels in"=w389, "data"=bool[] [FALSE, FALSE, FALSE, FALSE]) -> ()  [unwired: 11 in, 3 out]
                      }
                      frame #1 {
                        n208 = Wait (ms)(milliseconds to wait=u32 1000) -> ()  [unwired: 1 out]
                      }
                      frame #2 {
                        w391 = refnum<k21> "Polarity swtich 2"  # DAQmx Task Name
                        n209 = call-poly <vilib>:"DAQmx Write.vi"("task/channels in"=w391, "data"=bool[] [TRUE, FALSE, FALSE, TRUE]) -> ()  [unwired: 11 in, 3 out]
                      }
                    }
                  }
                }
              }
            }
          }
        }
        n210 = case shown="False" "Start switching 1" {
          tunnel: w326 -> [_ w449]
          tunnel: [FALSE w453] -> w325
          tunnel: w324 -> [_ w452]
          frame False {
            w446 = refnum<k21> "Polarity switch 1"  # DAQmx Task Name
            n211 = call-poly <vilib>:"DAQmx Write.vi"("task/channels in"=w446, "data"=bool[] [FALSE, FALSE, FALSE, FALSE]) -> ()  [unwired: 11 in, 3 out]
          }
          frame True {
            n212 = Multiply(x="Switching time 1 (s)", y=2.0) -> (x*y=w455:dbl)
            n213 = call "Elapsed Time"("Time Target (s)"=w455, "Reset"=w449) -> ("Elapsed Time (s)"=w450:dbl)  [unwired: 10 in, 7 out]
            "Present 1 (s)" <- w450
            n214 = Greater?(x="Switching time 1 (s)", y=w450) -> (0:w453:bool)
            n215 = Not Equal?(x=w452, y=w453) -> (x != y?=w451:bool)
            n216 = case shown="True" w453 {
              tunnel: w451 -> [w457 w463]
              frame False {
                n217 = case shown="True" w457 {
                  frame False {
                  }
                  frame True {
                    n218 = flat-sequence {
                      frame #0 {
                        w459 = refnum<k21> "Polarity switch 1"  # DAQmx Task Name
                        n219 = call-poly <vilib>:"DAQmx Write.vi"("task/channels in"=w459, "data"=bool[] [FALSE, FALSE, FALSE, FALSE]) -> ()  [unwired: 11 in, 3 out]
                      }
                      frame #1 {
                        n220 = Wait (ms)(milliseconds to wait=u32 1000) -> ()  [unwired: 1 out]
                      }
                      frame #2 {
                        w461 = refnum<k21> "Polarity switch 1"  # DAQmx Task Name
                        n221 = call-poly <vilib>:"DAQmx Write.vi"("task/channels in"=w461, "data"=bool[] [FALSE, TRUE, TRUE, FALSE]) -> ()  [unwired: 11 in, 3 out]
                      }
                    }
                  }
                }
              }
              frame True {
                n222 = case shown="True" w463 {
                  frame False {
                  }
                  frame True {
                    n223 = flat-sequence {
                      frame #0 {
                        w465 = refnum<k21> "Polarity switch 1"  # DAQmx Task Name
                        n224 = call-poly <vilib>:"DAQmx Write.vi"("task/channels in"=w465, "data"=bool[] [FALSE, FALSE, FALSE, FALSE]) -> ()  [unwired: 11 in, 3 out]
                      }
                      frame #1 {
                        n225 = Wait (ms)(milliseconds to wait=u32 1000) -> ()  [unwired: 1 out]
                      }
                      frame #2 {
                        w467 = refnum<k21> "Polarity switch 1"  # DAQmx Task Name
                        n226 = call-poly <vilib>:"DAQmx Write.vi"("task/channels in"=w467, "data"=bool[] [TRUE, FALSE, FALSE, TRUE]) -> ()  [unwired: 11 in, 3 out]
                      }
                    }
                  }
                }
              }
            }
          }
        }
        n227 = case shown="True" "Count down 1" {
          frame False {
          }
          frame True {
            n228 = local read "Sample waiting time 1 (min)"() -> (w401:dbl)
            n229 = Greater?(x=w401, y="Target wait time 1 (min)") -> (0:w399:bool)
            n230 = case shown="True" w399 {
              frame False {
              }
              frame True {
                w403 = FALSE ("Start switching")
                n231 = local write "Channel 1 control"(w403) -> ()
                n232 = local write "Count down 1"(w403) -> ()
                n233 = local write "Start switching 1"(w403) -> ()
                n234 = property on="Enable Output 1" class="Bool (strict)"("Val(Sgnl)"=w403) -> ()  [unwired: 2 in, 2 out]
                n235 = property on="Channel 2 SP (C)" class="DigNum (strict)"("Val(Sgnl)"=10.0 ("Value (Signaling)")) -> ()  [unwired: 2 in, 2 out]
              }
            }
          }
        }
        n236 = case shown="True" "Timing 2" {
          frame False {
            n237 = Get Date/Time In Seconds() -> (seconds since 1Jan1904=→"Start time 2":timestamp)
          }
          frame True {
            n238 = local read "Start time 2"() -> (w397:timestamp)
            n239 = Get Date/Time In Seconds() -> (seconds since 1Jan1904=w398:timestamp)
            "Current time 2" <- w398
            n240 = Subtract(x=w398, y=w397) -> (x-y=w395:dbl)
            n241 = Divide(x=w395, y=60.0) -> (x/y=→"Sample waiting time 2 (min)":dbl)
          }
        }
        n242 = case shown="True" "Count down 2" {
          frame False {
          }
          frame True {
            n243 = local read "Sample waiting time 2 (min)"() -> (w331:dbl)
            n244 = Greater?(x=w331, y="Target wait time 2 (min)") -> (0:w329:bool)
            n245 = case shown="True" w329 {
              frame False {
              }
              frame True {
                w333 = FALSE ("Start switching")
                n246 = local write "Channel 2 control"(w333) -> ()
                n247 = local write "Start switching 2"(w333) -> ()
                n248 = local write "Count down 2"(w333) -> ()
                n249 = property on="Enable Output 2" class="Bool (strict)"("Val(Sgnl)"=w333) -> ()  [unwired: 2 in, 2 out]
                n250 = property on="Channel 1 SP (C)" class="DigNum (strict)"("Val(Sgnl)"=10.0 ("Value (Signaling)")) -> ()  [unwired: 2 in, 2 out]
              }
            }
          }
        }
        n251 = Wait (ms)(milliseconds to wait=u32 500) -> ()  [unwired: 1 out]
      }
    }
    frame #2 {
      w469 = refnum<k21> "Polarity swtich 2"  # DAQmx Task Name
      w475 = refnum<k21> "Polarity switch 1"  # DAQmx Task Name
      n252 = local read "J-KEM COM"() -> (w473:refnum<visa-resource-name>)
      n253 = local read "DC power supply"() -> (w471:refnum<visa-resource-name>)
      n254 = call <instrlib>:"Close.vi"("VISA resource name"=w471) -> ()  [unwired: 10 in, 1 out]
      n255 = local write "stop"(FALSE ("stop")) -> ()
      n256 = call-poly <vilib>:"DAQmx Write.vi"("task/channels in"=w475, "data"=bool[] [FALSE, FALSE, FALSE, FALSE]) -> ()  [unwired: 11 in, 3 out]
      n257 = call-poly <vilib>:"DAQmx Write.vi"("task/channels in"=w469, "data"=bool[] [FALSE, FALSE, FALSE, FALSE]) -> ()  [unwired: 11 in, 3 out]
      n258 = call <instrlib>:"Close.vi"("VISA resource name"=w473) -> ()  [unwired: 10 in, 1 out]
    }
  }
